vi "TestExec.Eq List to Table.vi"(1 "Eq List":T1[](array[typedef])) -> (0 "Table":string[][](table))   [LabVIEW 2018]
uses:
  Common/Utils/Results/Result XML/TestResult.HW Item.ctl
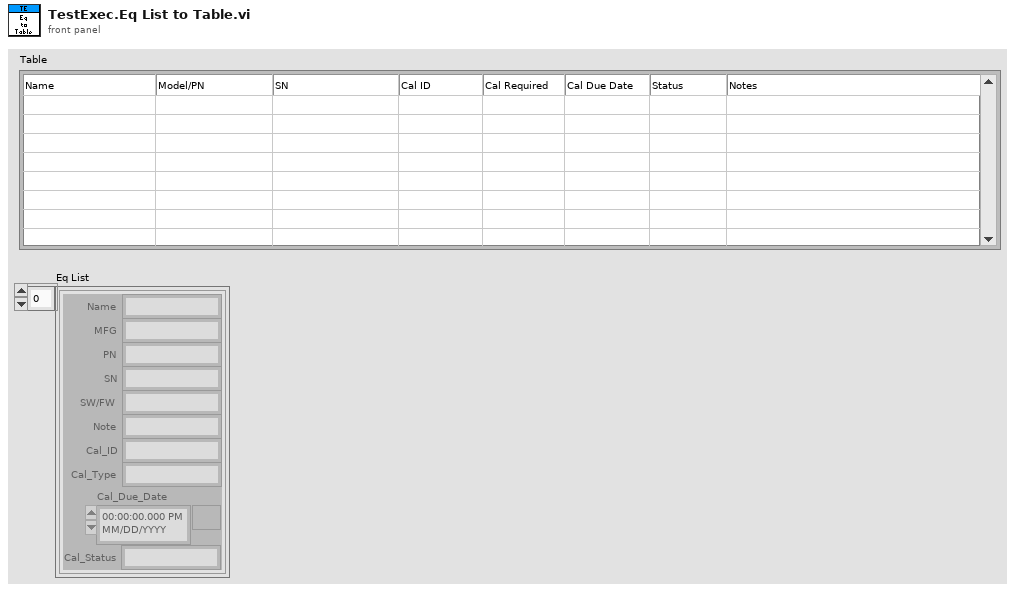
[diagram p1: front panel]
types:
  T1 = typedef "TestResult.HW Item.ctl" = cluster{"Name":string, "MFG":string, "PN":string, "SN":string, "SW/FW":string, "Note":string, "Cal_ID":string, "Cal_Type":string, "Cal_Due_Date":timestamp, "Cal_Status":string}
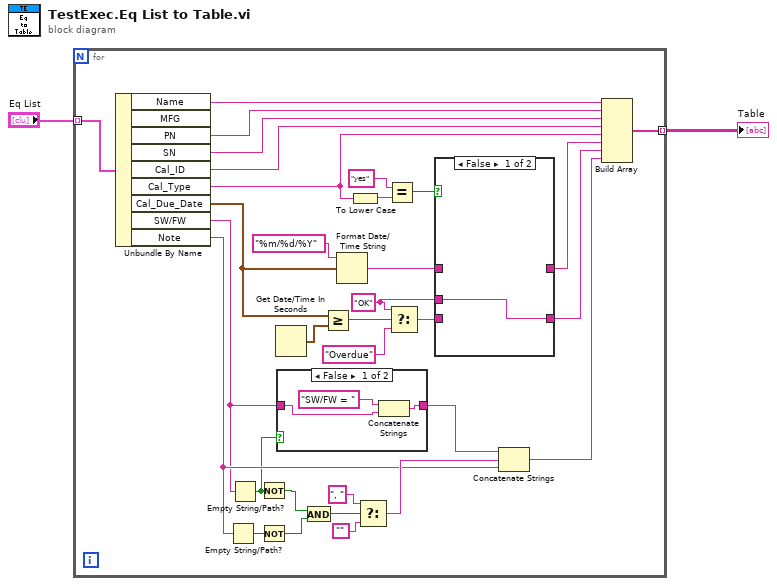
[diagram p0: block diagram]
diagram:
  n1 = for {
    tunnel: "Eq List" -> [w34] mode=indexing
    tunnel: [w10] -> w1 mode=indexing
    w9 = "OK"
    n2 = Unbundle By Name(w34) -> ("Name"=w33:string, "PN"=w32:string, "SN"=w31:string, "Cal_ID"=w25:string, "Cal_Type"=w24:string, "Cal_Due_Date"=w21:timestamp, "SW/FW"=w4:string, "Note"=w26:string)  [unwired: 1 out]
    n3 = Empty String/Path?(string/path=w26) -> (empty?=w8:bool)
    n4 = Empty String/Path?(string/path=w4) -> (empty?=w5:bool)
    n5 = Not(x=w5) -> (.not. x?=w7:bool)
    n6 = Not(x=w8) -> (.not. x?=w6:bool)
    n7 = Get Date/Time In Seconds() -> (seconds since 1Jan1904=w20:timestamp)
    n8 = case shown="False" w5 {
      tunnel: w4 -> [w35 w38]
      tunnel: [w36 w38] -> w3
      frame False {
        n9 = Concatenate Strings("SW/FW = ", w35) -> (w36:string)
      }
      frame True {
      }
    }
    n10 = And(x=w7, y=w6) -> (x .and. y?=w30:bool)
    n11 = Greater Or Equal?(x=w21, y=w20) -> (x >= y?=w18:bool)
    n12 = Format Date/Time String(time format string (%c)="%m/%d/%Y", seconds (now)=w21) -> (date/time string=w16:string)  [unwired: 1 in]
    n13 = To Lower Case(string=w24) -> (all lower case string=w23:string)
    n14 = Select(t=", ", s=w30, f="") -> (s? t:f=w27:string)
    n15 = Equal?(x="yes", y=w23) -> (x = y?=w14:bool)
    n16 = Select(t=w9, s=w18, f="Overdue") -> (s? t:f=w15:string)
    n17 = case shown="False" w14 {
      tunnel: w16 -> [_ w41]
      tunnel: w15 -> [_ w40]
      tunnel: [_ w41] -> w13
      tunnel: [w39 w40] -> w12
      tunnel: w9 -> [w39 _]
      frame False {
      }
      frame True {
      }
    }
    n18 = Concatenate Strings(w3, w27, w26) -> (w11:string)
    n19 = Build Array(w33, w32, w31, w25, w24, w13, w12, w11) -> (w10:string[])
  }
  "Table" <- w1
